vi "Output.vi"(8 "error in (no error)":errorcluster, 9 "Enable Output (T: Enable)":bool=TRUE, 10 "Channel (0: Channel 1)":i32(ring) items=["", "Channel 1", "Channel 2"], 11 "VISA Refnum in":refnum<visa-resource-name>) -> (0 "error out":errorcluster, 3 "VISA Refnum out":refnum<visa-resource-name>)   [LabVIEW 2023]
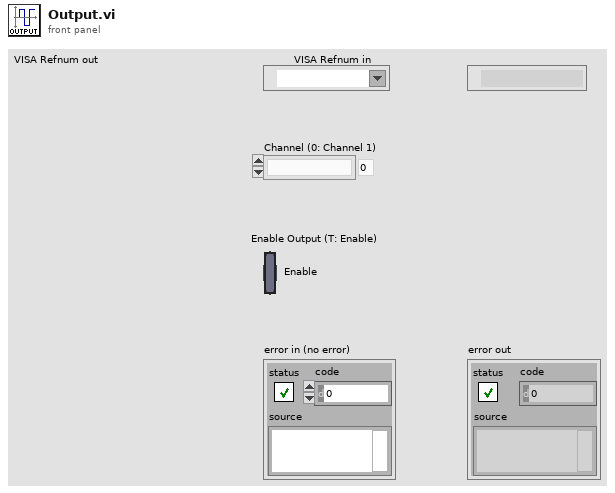
[diagram p1: front panel]
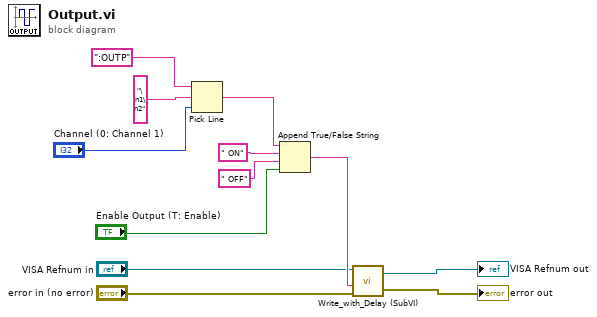
[diagram p0: block diagram]
diagram:
  n1 = Pick Line(string ("")=":OUTP", multi-line string="\n1\n2", line index="Channel (0: Channel 1)") -> (output string=w7:string)
  n2 = Append True/False String(1:"Enable Output (T: Enable)", 2:" OFF" ("true string"), 3:" ON" ("true string"), 4:w7) -> (0:w5:string)
  n3 = call "Write_with_Delay (SubVI).vi"("error in (no error)"="error in (no error)", "Command"=w5, "VISA Refnum in"="VISA Refnum in") -> ("error out"=→"error out":errorcluster, "VISA Refnum out"=→"VISA Refnum out":refnum<visa-resource-name>)  [unwired: 1 in]
